vi "Handle Command.vi"(8 "error in (no error)":errorcluster, 9 "Data":variant, 10 "Command":string, 11 "Instrument.VoltageSource in":refnum<class "Instrument.VoltageSource.lvclass">) -> (0 "error out":errorcluster, 1 "Processed Data":variant, 2 "Command":string, 3 "Instrument.VoltageSource out":refnum<class "Instrument.VoltageSource.lvclass">)   [LabVIEW 2016, in "Instrument.VoltageSource.lvclass"]
uses:
  Instrument.VoltageSource.lvclass
  Instrument.VoltageSource.lvclass/Instrument.VoltageSource.ctl
  <vilib>/DAQmx/write.llb/DAQmx Write (Analog DBL 1Chan 1Samp).vi
  <vilib>/DAQmx/miscellaneous.llb/DAQmx Fill In Error Info.vi
  <userlib>/LevyLab/Levylab Instruments/Instrument Types/VSource/Instrument.VSource.lvclass
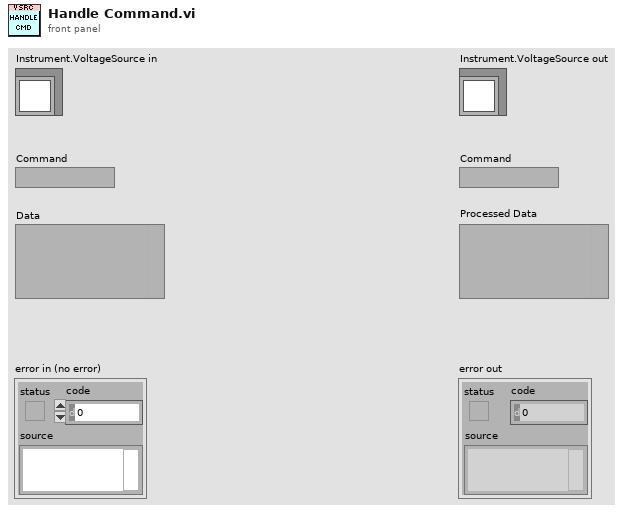
[diagram p1: front panel]
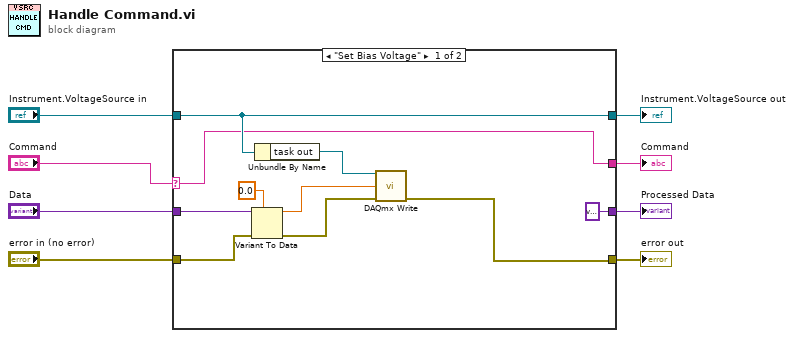
[diagram p0: block diagram]
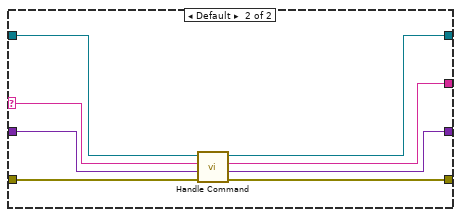
[diagram p2: hidden frame]
diagram:
  n1 = case shown="\"Set Bias Voltage\"" "Command" {
    selector: "Command" -> [w10 w19]
    tunnel: [w13 w26] -> w8
    tunnel: [variant ("Processed Data") w25] -> w7
    tunnel: [w10 w24] -> w6
    tunnel: [w11 w23] -> w5
    tunnel: "error in (no error)" -> [w14 w22]
    tunnel: "Data" -> [w18 w21]
    tunnel: "Instrument.VoltageSource in" -> [w11 w20]
    frame "Set Bias Voltage" {
      n2 = Variant To Data(error in=w14, type=0.0 ("data"), Variant=w18) -> (data=w16:dbl, error out=w15:errorcluster)
      n3 = Unbundle By Name(w11) -> ("task out"=w12:refnum<k21>)
      n4 = call-poly <vilib>:"DAQmx Write.vi"("task/channels in"=w12, "data"=w16, "error in"=w15) -> ("error out"=w13:errorcluster)  [unwired: 10 in, 2 out]
    }
    frame Default {
      n5 = call-parent "Handle Command.vi"("error in (no error)"=w22, "Data"=w21, "Command"=w19, "Instrument in"=w20) -> ("error out"=w26:errorcluster, "Processed Data"=w25:variant, "Command"=w24:string, "Instrument out"=w23:refnum<class "Instrument.VoltageSource.lvclass">)  [unwired: 4 in]
    }
  }
  "error out" <- w8
  "Instrument.VoltageSource out" <- w5
  "Processed Data" <- w7
  "Command" <- w6
